vi "Read SA Pin.vi"(8 "error in (no error)":errorcluster, 11 "Insertion Loss in":refnum<class "Insertion Loss.lvclass">=refnum) -> (0 "error out":errorcluster, 2 "SA Pin":string, 3 "Insertion Loss out":refnum<class "Insertion Loss.lvclass">)   [LabVIEW 2016, in "SeqAuto Evaluations.lvlib" / "Insertion Loss.lvclass"]
uses:
  Insertion Loss.lvclass
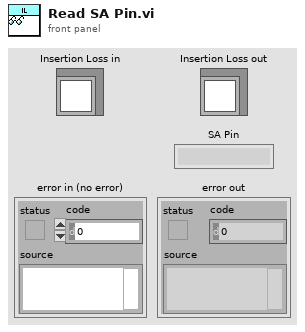
[diagram p1: front panel]
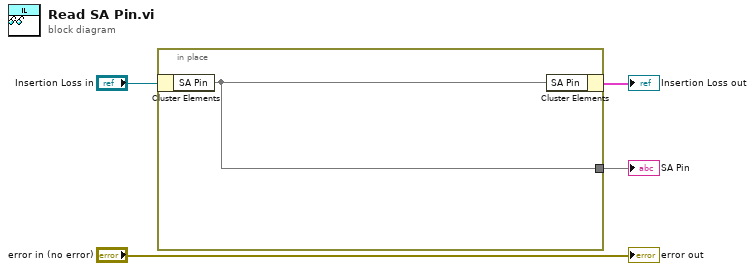
[diagram p0: block diagram]
diagram:
  n1 = in-place {
    in-place-border: [w5] -> w3
    n2 = in-place-cluster #1("Insertion Loss in") -> ("SA Pin"=w5)
    n3 = in-place-cluster #1("SA Pin"=w5) -> (→"Insertion Loss out":cluster{})
  }
  "SA Pin" <- w3
  "error out" <- "error in (no error)"
